vi "Tosca-Start TTL Thread.vi"(0 "TTLDevice":refnum<class "TTLControlledDevice.lvclass">, 2 "Thread Notifier":refnum<notifier>, 7 "Control Queue":refnum<queue>, 11 "error in (no error)":errorcluster) -> (15 "error out":errorcluster)   [LabVIEW 2020]
uses:
  Device Classes/Base Class/TTLControlledDevice.lvclass
  Control Classes/Base Class/TTLController.lvclass
panel:
  in  "First":bool
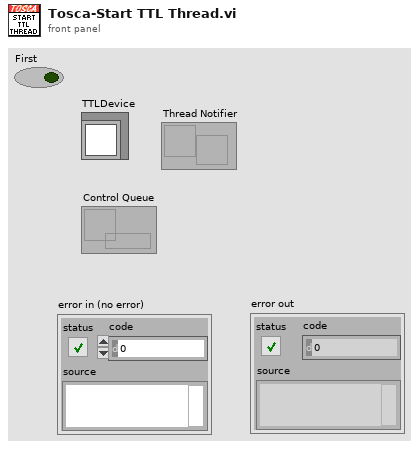
[diagram p1: front panel]
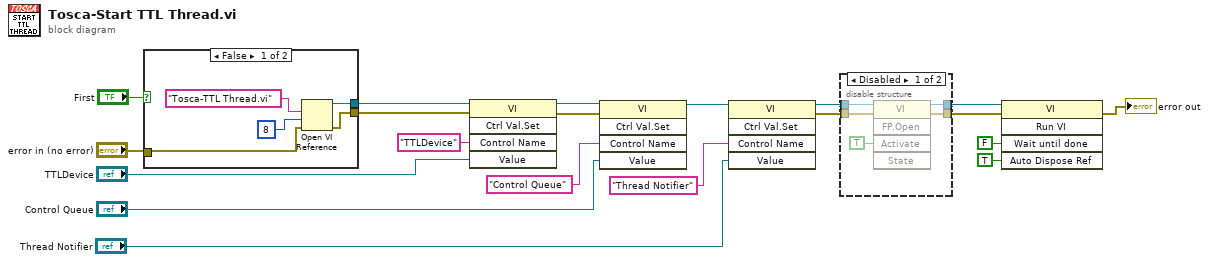
[diagram p0: block diagram]
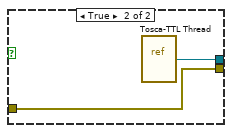
[diagram p2: hidden frame]
diagram:
  n1 = case shown="False" "First" {
    tunnel: "error in (no error)" -> [w25 w27]
    tunnel: [w24 w27] -> w14
    tunnel: [w22 w26] -> w2
    frame False {
      n2 = Open VI Reference(vi path="Tosca-TTL Thread.vi", options=8, error in (no error)=w25) -> (vi reference=w22:refnum<vi>, error out=w24:errorcluster)  [unwired: 3 in]
    }
    frame True {
      n3 = vi-ref "Tosca-TTL Thread.vi"() -> (w26:refnum<vi>)
    }
  }
  n4 = invoke class="VI" method="Ctrl Val.Set"(reference=w2, error in=w14, "Control Name"="TTLDevice", "Value"="TTLDevice") -> (reference out=w19:refnum<vi>, error out=w18:errorcluster)  [unwired: 1 in, 3 out]
  n5 = invoke class="VI" method="Ctrl Val.Set"(reference=w19, error in=w18, "Control Name"="Control Queue", "Value"="Control Queue") -> (reference out=w7:refnum<vi>)  [unwired: 1 in, 4 out]
  n6 = invoke class="VI" method="Ctrl Val.Set"(reference=w7, "Control Name"="Thread Notifier", "Value"="Thread Notifier") -> (reference out=w6:refnum<vi>, error out=w3:errorcluster)  [unwired: 2 in, 3 out]
  n7 = disable-structure shown="Disabled" {
    disable-tunnel: [w32 w34] -> w9
    disable-tunnel: [w31 w33] -> w8
    disable-tunnel: w6 -> [w29 w34]
    disable-tunnel: w3 -> [w28 w33]
    frame Disabled {
      n8 = invoke class="VI" method="FP.Open"(reference=w29, error in=w28, "Activate"=TRUE ("Activate?")) -> (reference out=w32:refnum<vi>, error out=w31:errorcluster)  [unwired: 2 in, 3 out]
    }
    frame Enabled {
    }
  }
  n9 = invoke class="VI" method="Run VI"(reference=w9, error in=w8, "Wait until done"=FALSE ("Wait Until Done"), "Auto Dispose Ref"=TRUE ("Auto Dispose Reference")) -> (error out=→"error out":errorcluster)  [unwired: 1 in, 4 out]
